vi "Check Versions.vi"(0 "Register Buses":T1[](array[typedef]), 11 "error in":errorcluster) -> (4 "Register Buses (out)":T1[](array[typedef]), 15 "error out":errorcluster)   [LabVIEW 2014, in "ni579x Synchronization v2 Host.lvlib"]
uses:
  <instrlib>/ni579x/Synchronization/v2/Host/ni579x Synchronization v2 Host.lvlib
  <instrlib>/_niInstr/Register Bus/v0/Host/Public/Register Bus Session.ctl
  <instrlib>/_niInstr/Register Bus/v0/Host/Private/Session Data.ctl
  <instrlib>/_niInstr/Register Bus/v0/Host/Public/Register Read Request.ctl
  <instrlib>/ni579x/Synchronization/v2/Shared/ni579x Synchronization Register Addresses.ctl
  <instrlib>/ni579x/Config/v2/Shared/Types/ni579x Register Bus Subsystem ID.ctl
  <vilib>/Utility/error.llb/Error Cluster From Error Code.vi
  <vilib>/ErrorRing/Error Ring.xnode
  <instrlib>/ni579x/Config/v2/Shared/ni579x Config v2 Shared.lvlib
  <instrlib>/_niInstr/Register Bus/v0/Host/niInstr Register Bus v0 Host.lvlib
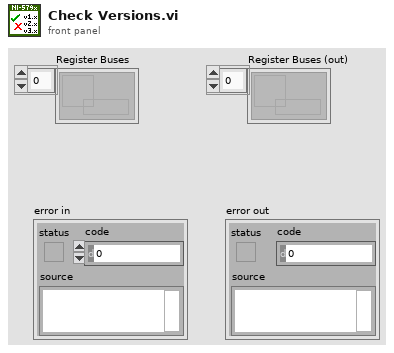
[diagram p1: front panel]
types:
  T1 = typedef "niInstr Register Bus v0 Host.lvlib/Register Bus Session.ctl" = refnum<queue>
  T2 = typedef "ni579x Config v2 Shared.lvlib/ni579x Register Bus Subsystem ID.ctl" = u8
  T3 = typedef "ni579x Synchronization Register Addresses.ctl" = enum16{"Signature", "Current Version", "Oldest Compatible Version", "Scratch Register", "sync.master", "sync.meas.enable", "sync.meas.ready", "sync.meas.arm", "sync.meas.valid", "sync.meas.value", "sync.cptr.adjust", "sync.cptr.period", "sync.meas.oversample factor"}
  T4 = typedef "niInstr Register Bus v0 Host.lvlib/Register Read Request.ctl" = cluster{"subsystem":u8, "address":u16}
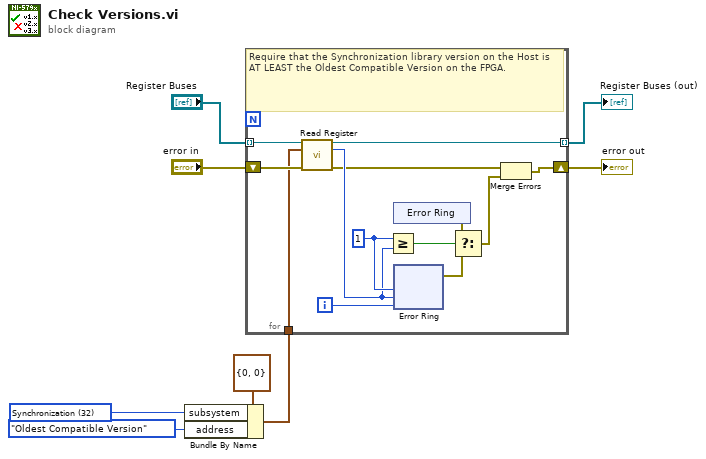
[diagram p0: block diagram]
diagram:
  w2 = T2 32 items=["FAM Register Operation"=0, "User Command"=16, "Synchronization"=32] ("Subsystem ID")
  n1 = Bundle By Name(cluster=T4 {"subsystem"=0, "address"=0} ("register read request"), "subsystem"=w2, "address"=ni579x_Synchronization_Register_Addresses."Oldest Compatible Version" ("Synchronization Registers")) -> (w8:T4)
  n2 = for {
    tunnel: "Register Buses" -> [w20] mode=indexing
    shift-right: [w11] -> w6
    shift-left: "error in" -> [w21]
    tunnel: w8 -> [w19]
    tunnel: [w10] -> w5 mode=indexing
    i -> [w13]
    w15 = u32 1 ("data")
    # "Require that the Synchronization library version on the Host is AT LEAST the Oldest Compatible Version on the FPGA."
    n3 = call <instrlib>:"Read Register.vi"("session in"=w20, "register read request"=w19, "error in"=w21) -> ("session out"=w10:T1, "data"=w14:u32, "error out"=w12:errorcluster)  [unwired: 10 in]
    n4 = Greater Or Equal?(x=w15, y=w14) -> (x >= y?=w9:bool)
    n5 = xnode "Error Ring"() -> ("error out"=w16:errorcluster)
    n6 = xnode "Error Ring"("parameter 0"=w15, "parameter 1"=w14, "parameter 2"=w13) -> ("error out"=w18:errorcluster)
    n7 = Select(t=w16, s=w9, f=w18) -> (s? t:f=w17:errorcluster)
    n8 = Merge Errors(w12, w17) -> (w11:errorcluster)
  }
  "error out" <- w6
  "Register Buses (out)" <- w5
